vi "SEQ Lossy Enqueue.vi"(8 "error in (no error)":errorcluster, 10 "Setting":T1, 11 "Queue Name":string) -> (0 "error out":errorcluster)   [LabVIEW 2019, in "ADLINK Motion Card.lvlib"]
uses:
  ADLINK Motion Card.lvlib
  SEQ Data.ctl
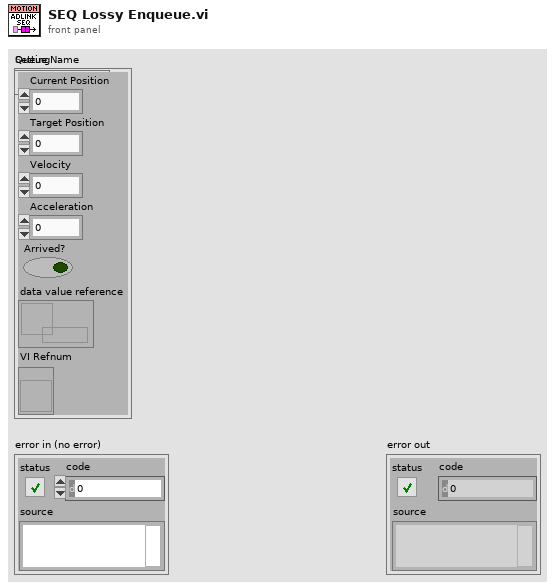
[diagram p1: front panel]
types:
  T1 = typedef "ADLINK Motion Card.lvlib/SEQ Data.ctl" = cluster{"Current Position":dbl, "Target Position":dbl, "Velocity":dbl, "Acceleration":dbl, "Arrived?":bool, "data value reference":refnum<data-value>, "VI Refnum":refnum<vi>}
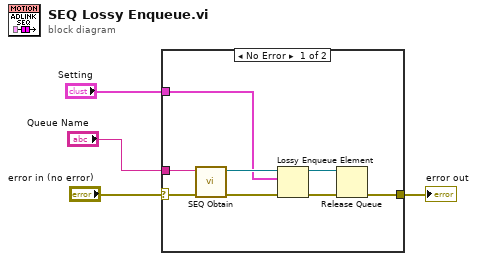
[diagram p0: block diagram]
diagram:
  n1 = case shown="No Error" "error in (no error)" {
    selector: "error in (no error)" -> [w6 w13]
    tunnel: "Queue Name" -> [w12 _]
    tunnel: "Setting" -> [w9 _]
    tunnel: [w5 w13] -> w1
    frame No Error {
      n2 = call "SEQ Obtain.vi"("error in (no error)"=w6, "Queue Name"=w12) -> ("error out"=w10:errorcluster, "queue out"=w11:refnum<queue>)  [unwired: 8 in]
      n3 = Lossy Enqueue Element(queue=w11, element=w9, error in (no error)=w10) -> (queue out=w8:refnum<queue>, error out=w7:errorcluster)  [unwired: 2 out]
      n4 = Release Queue(queue=w8, error in (no error)=w7) -> (error out=w5:errorcluster)  [unwired: 1 in, 2 out]
    }
    frame Error {
    }
  }
  "error out" <- w1
